vi "Get Digital Patterns - Multi FPGA.vi"(8 "error in (no error)":errorcluster, 10 "RIO Address":string, 11 "Item Ref in":T1 format="%.0x") -> (0 "error out":errorcluster, 1 "references":T1[](array[typedef]) format="%.0x", 2 "Patterns":T2[](array[typedef]))   [LabVIEW 2015, in "Engine Simulation Toolkit System Explorer.lvlib"]
uses:
  Engine Simulation Toolkit System Explorer.lvlib
  <vilib>/NI Veristand/Custom Device API/Custom Device Item Ref.ctl
  Digital Pattern.ctl
  Digital Pattern Base.ctl
  Digital Pattern Remove Edge.ctl
  Digital Pattern Add Pulse.ctl
  <vilib>/NI Veristand/Custom Device API/Custom Device API.lvlib
panel:
  # "If empty, return digital patterns\nfor all RIOs"
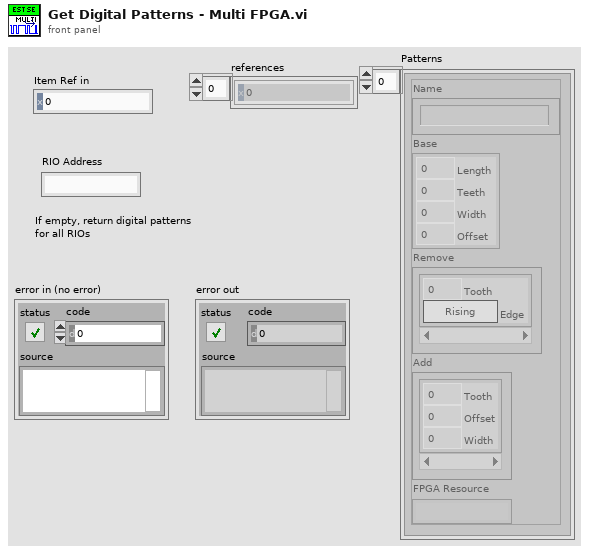
[diagram p1: front panel]
types:
  T1 = typedef "Custom Device API.lvlib/Custom Device Item Ref.ctl" = u64
  T2 = typedef "Engine Simulation Toolkit System Explorer.lvlib/Digital Pattern.ctl" = cluster{"Name":string, "Base":T3, "Remove":T4[], "Add":T5[], "FPGA Resource":string}
  T3 = typedef "Engine Simulation Toolkit System Explorer.lvlib/Digital Pattern Base.ctl" = cluster{"Length":dbl, "Teeth":u16, "Width":dbl, "Offset":dbl}
  T4 = typedef "Engine Simulation Toolkit System Explorer.lvlib/Digital Pattern Remove Edge.ctl" = cluster{"Tooth":u16, "Edge":bool}
  T5 = typedef "Engine Simulation Toolkit System Explorer.lvlib/Digital Pattern Add Pulse.ctl" = cluster{"Tooth":u16, "Offset":dbl, "Width":dbl}
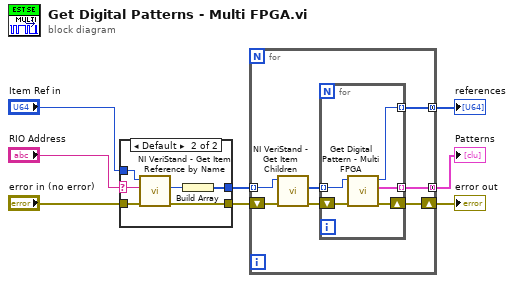
[diagram p0: block diagram]
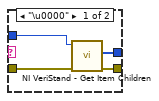
[diagram p2: hidden frame]
diagram:
  n1 = case shown="Default" "RIO Address" {
    selector: "RIO Address" -> [_ w13]
    tunnel: [w12 w17] -> w1
    tunnel: "error in (no error)" -> [w11 w15]
    tunnel: [w10 w16] -> w3
    tunnel: "Item Ref in" -> [w9 w14]
    frame "\u0000" {
      n2 = call <vilib>:"NI VeriStand - Get Item Children.vi"("error in (no error)"=w11, "Item Ref in"=w9) -> ("error out"=w10:errorcluster, "Child Refs"=w12:T1[])  [unwired: 6 in, 2 out]
    }
    frame Default {
      n3 = call <vilib>:"NI VeriStand - Get Item Reference by Name.vi"("error in (no error)"=w15, "Item Name"=w13, "Parent Ref in"=w14) -> ("error out"=w16:errorcluster, "Item Ref"=w18:T1)  [unwired: 5 in, 2 out]
      n4 = Build Array(w18) -> (w17:T1[])
    }
  }
  n5 = for {
    tunnel: [w24] -> w7 mode=concatenating
    tunnel: [w21] -> w6 mode=concatenating
    tunnel: w1 -> [w19] mode=indexing
    shift-right: [w25] -> w8
    shift-left: w3 -> [w20]
    n6 = call <vilib>:"NI VeriStand - Get Item Children.vi"("error in (no error)"=w20, "Item Ref in"=w19) -> ("error out"=w23:errorcluster, "Child Refs"=w22:T1[])  [unwired: 6 in, 2 out]
    n7 = for {
      shift-right: [w28] -> w25
      shift-left: w23 -> [w30]
      tunnel: [w27] -> w24 mode=indexing
      tunnel: w22 -> [w29] mode=indexing
      tunnel: [w26] -> w21 mode=indexing
      n8 = call "Get Digital Pattern - Multi FPGA.vi"("error in (no error)"=w30, "Item Ref in"=w29) -> ("error out"=w28:errorcluster, "EPT Pattern"=w27:T2, "Item Ref out"=w26:T1)  [unwired: 7 in]
    }
  }
  "error out" <- w8
  "Patterns" <- w7
  "references" <- w6
